vi "Calib_General_Setup.vi"(0 "Ref Instrument type":T1=enum."Generic Polynomial", 1 "Requested No of samples":i32=128 min=0 step=1, 2 "Sampling rate (Hz)":sgl=1000.0 format="%.2f", 5 "2nd ref instrument":T2={"2nd Ref type"=enum."LDA", "2nd inst present"=TRUE}, 9 "Temp":dbl=20.0 format="%.1f", 12 "Abs Press (mbar)":dbl=1005.0 format="%.2f") -> (8 "Output string":string, 10 "LDA Data":bool)   [LabVIEW 2022 SP3]
uses:
  Controls/Ref_Inst_type.ctl
  Controls/Analysis_info_cluster.ctl
  Controls/Inst_type.ctl
  Controls/Instrument_Array.ctl
  Controls/channelState.ctl
  Controls/Graph_Type.ctl
  Globals/Meas_global.vi
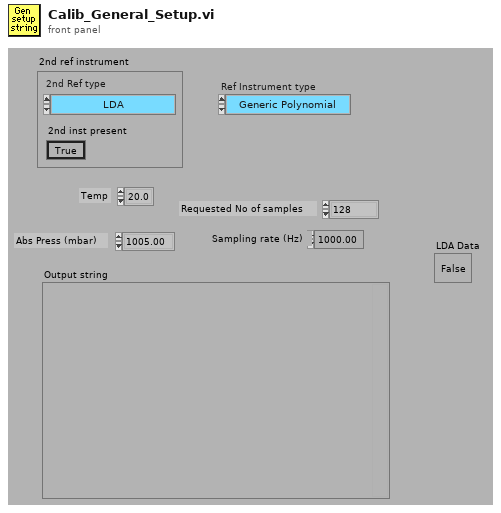
[diagram p1: front panel]
types:
  T1 = typedef "Ref_Inst_type.ctl" = enum16{"Propellor anemometer", "Pressure Transducer", "Raw voltage", "Pitot-static tube", "Generic Linear", "Generic Polynomial", "Thermocouple", "LDA", "Enter Value", "ADAM Channel"}
  T2 = cluster{"2nd Ref type":T1, "2nd inst present":bool}
  T3 = typedef "Analysis_info_cluster.ctl" = cluster{"Colour":u32, "Inst type":T4, "Inst name":string, "Symbol":string, "Code name":string, "Extra Info":string, "Inst Array":T5, "U":dbl, "u^2":dbl, "u^3":dbl, "u^4":dbl, "Skew_u":dbl, "Kurt_u":dbl, "Sd Error in Mean":dbl, "% u'/U":dbl, "X":dbl, "Y":dbl, "Z":dbl, "Timescale integral Estimate":dbl, "Sd Error in Variance":dbl, "Calib File":path, "Calib Constants":dbl[], "Output Position":bool, "Stats":enum16{"None", "Basic", "Full"}, "Av Sampling Rate":dbl, "Av No of Samples":dbl, "Total Meas Time (s)":dbl, "OrigChName":string, "Max value":dbl, "Min value":dbl, "Req Sample Rate Hz":dbl, "Sync Delay Time (s)":dbl, "Ch No":i16, "Device":string, "Use Latest Calib":bool, "Port":string, "Metadata Ch Names":string[], "Metadata Ch Values":string[], "Label":string, "chState":T6, "Point Drift":dbl, "inputConfig":string}
  T4 = typedef "Inst_type.ctl" = enum16{"Raw voltage", "Raw with zero offsetting", "Propeller anemometer", "Pressure Transducer", "Pitot-static tube", "Hot wire", "Cross wire 1", "Cross wire 2", "Generic Linear", "Generic Polynomial", "Generic BackPoly", "Fast FID", "Thermocouple", "Cold wire", "Pulsed Wire", "LDA Vel", "LDA Tran time", "LDA Arr time", "Microphone"}
  T5 = typedef "Instrument_Array.ctl" = enum16{"PWA", "LDA", "Analogue"}
  T6 = typedef "channelState.ctl" = enum32{"No Selection", "Solo", "Mute"}
  T7 = typedef "Graph_Type.ctl" = enum16{"Show no graph", "Voltage trace", "Velocity trace", "Vel histogram", "Spectrum", "f.E(f) v Log f", "Auto-Corr"}
  T8 = cluster{"Plot 1":u16, "Plot 2":u16, "Save graph":u16, "Plot Type":T7}
  T9 = enum16{"From String to Cluster", "From Cluster to String"}
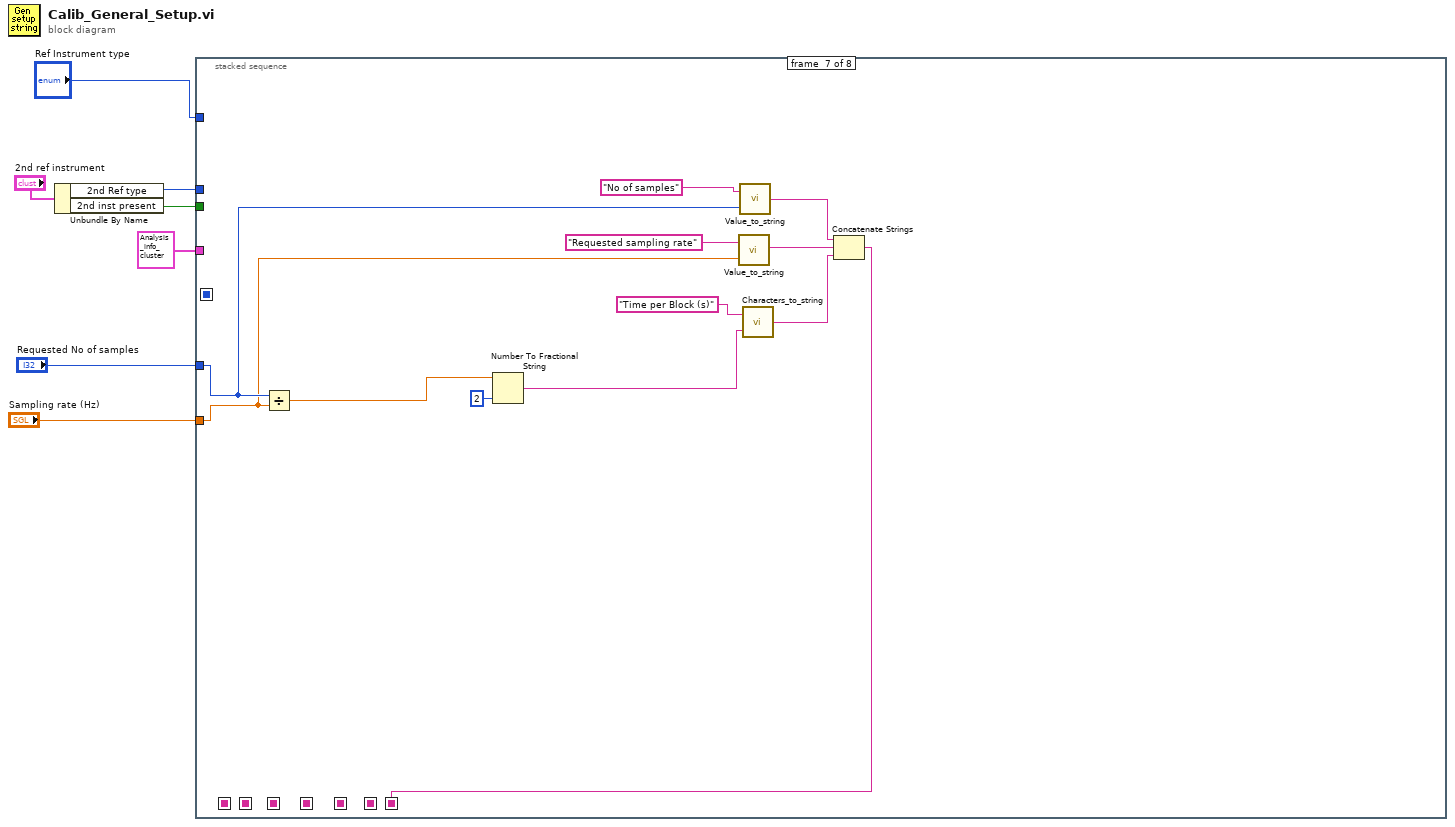
[diagram p0: block diagram]
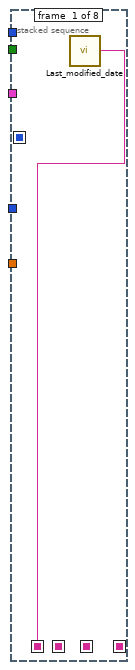
[diagram p2: hidden frame]
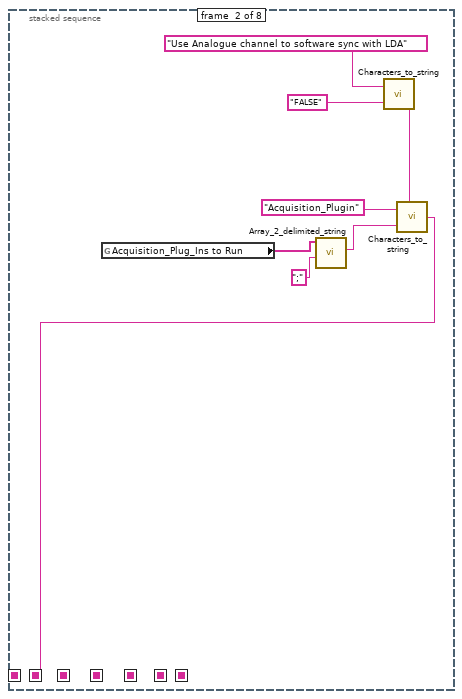
[diagram p3: hidden frame]
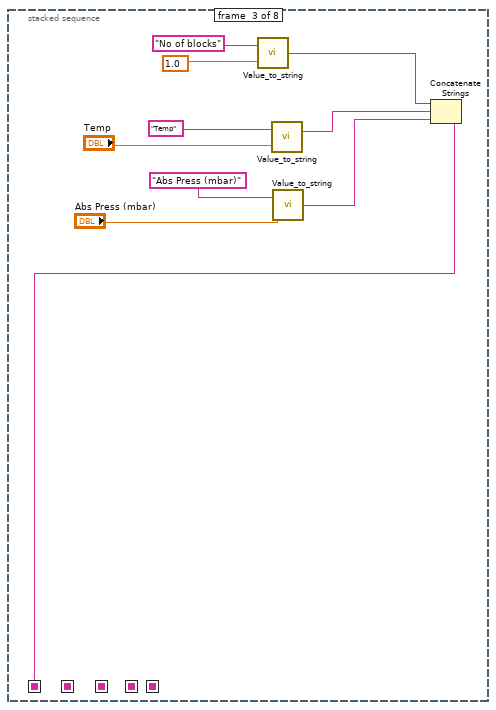
[diagram p4: hidden frame]
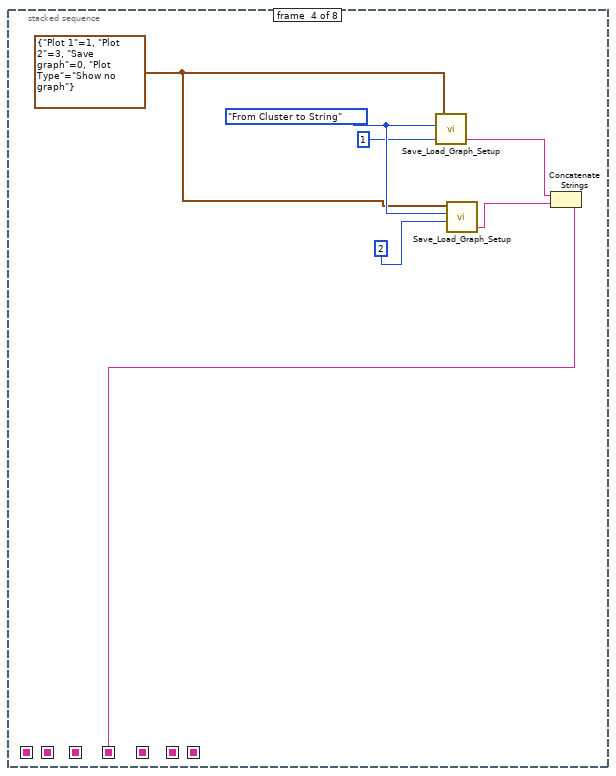
[diagram p5: hidden frame]
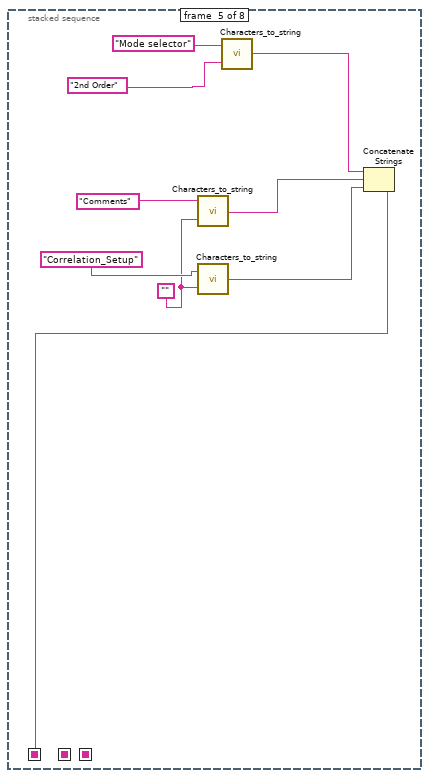
[diagram p6: hidden frame]
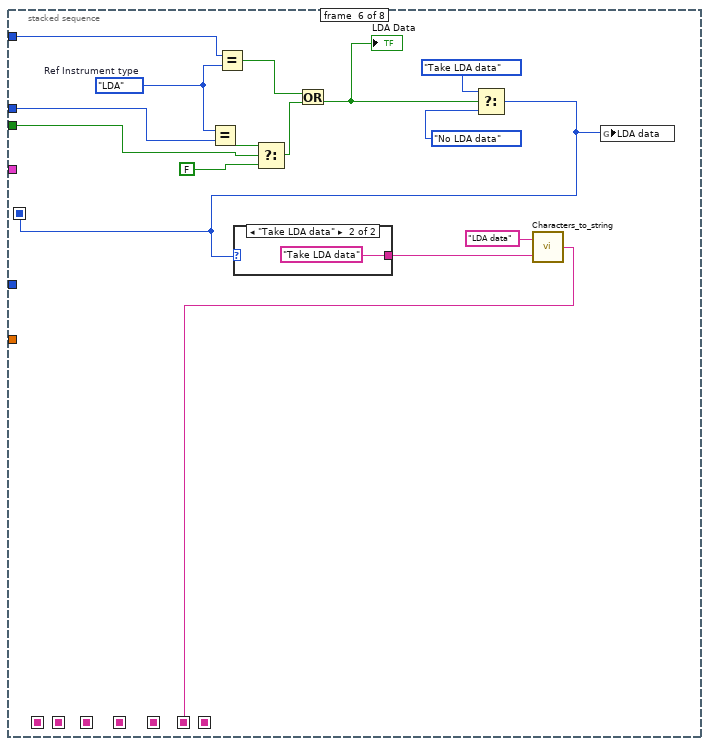
[diagram p7: hidden frame]
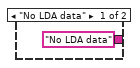
[diagram p8: hidden frame]
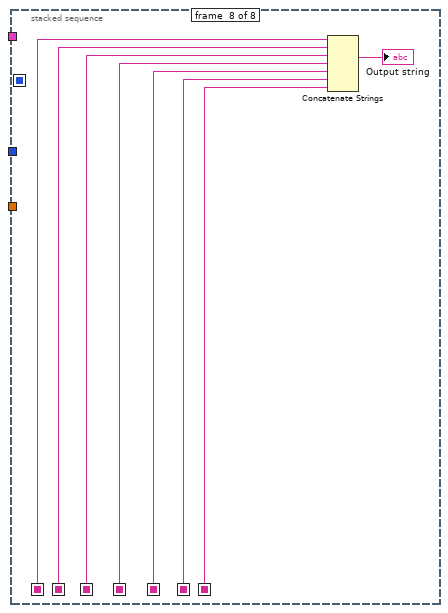
[diagram p9: hidden frame]
diagram:
  n1 = Unbundle By Name("2nd ref instrument") -> ("2nd Ref type"=w5:T1, "2nd inst present"=w4:bool)
  n2 = stacked-sequence {
    seq-local: [_ _ w25 _ _ _ _ _] -> [_ _ _ _ _ _ _ w79]
    seq-local: [_ w9 _ _ _ _ _ _] -> [_ _ _ _ _ _ _ w78]
    seq-local: [_ _ _ _ _ w55 _ _] -> [_ _ _ _ _ _ _ w74]
    seq-local: [_ _ _ _ _ _ w60 _] -> [_ _ _ _ _ _ _ w73]
    seq-local: [_ _ _ w28 _ _ _ _] -> [_ _ _ _ _ _ _ w76]
    seq-local: [_ _ _ _ w37 _ _ _] -> [_ _ _ _ _ _ _ w75]
    seq-local: [w8 _ _ _ _ _ _ _] -> [_ _ _ _ _ _ _ w72]
    seq-local: [_ _ _ _ _ w48 _ _] -> [_ _ _ _ _ _ _ _]
    tunnel: T3 {"Colour"=0, "Inst type"=enum."Pitot-static tube", "Inst name"="Manometer voltage", "Symbol"="U", "Code name"="", "Extra Info"="U", "Inst Array"=enum."PWA", "U"=0.0, "u^2"=0.0, "u^3"=0.0, "u^4"=0.0, "Skew_u"=0.0, "Kurt_u"=0.0, "Sd Error in Mean"=0.0, "% u'/U"=0.0, "X"=0.0, "Y"=0.0, "Z"=0.0, "Timescale integral Estimate"=0.0, "Sd Error in Variance"=0.0, "Calib File"=path "", "Calib Constants"=[], "Output Position"=FALSE, "Stats"=enum."None", "Av Sampling Rate"=0.0, "Av No of Samples"=0.0, "Total Meas Time (s)"=0.0, "OrigChName"="", "Max value"=0.0, "Min value"=0.0, "Req Sample Rate Hz"=0.0, "Sync Delay Time (s)"=0.0, "Ch No"=0, "Device"="", "Use Latest Calib"=FALSE, "Port"="", "Metadata Ch Names"=[], "Metadata Ch Values"=[], "Label"="", "chState"=enum."Solo", "Point Drift"=0.0, "inputConfig"=""} -> [_ _ _ _ _ _ _ _]
    tunnel: "Ref Instrument type" -> [_ _ _ _ _ w45 _ _]
    tunnel: w5 -> [_ _ _ _ _ w44 _ _]
    tunnel: w4 -> [_ _ _ _ _ w43 _ _]
    tunnel: "Requested No of samples" -> [_ _ _ _ _ _ w65 _]
    tunnel: "Sampling rate (Hz)" -> [_ _ _ _ _ _ w64 _]
    frame #0 {
      n3 = call "Last_modified_date.vi"() -> ("concatenatedRevisions"=w8:string)  [unwired: 1 in, 1 out]
    }
    frame #1 {
      n4 = global read "Meas_global.vi" "Acquisition_Plug_Ins to Run"() -> (w12:string[])
      n5 = call "Array_2_delimited_string.vi"("delimiter (Tab)"=";", "Array of Strings"=w12) -> ("delimited string"=w13:string)  [unwired: 9 in]
      n6 = call "Characters_to_string.vi"("Characters to write"="FALSE", "Label for characters"="Use Analogue channel to software sync with LDA") -> ("Output string"=w10:string)  [unwired: 1 in]
      n7 = call "Characters_to_string.vi"("stringIn"=w10, "Characters to write"=w13, "Label for characters"="Acquisition_Plugin") -> ("Output string"=w9:string)
    }
    frame #2 {
      n8 = call "Value_to_string.vi"("Value"=1.0, "Label for value"="No of blocks") -> ("Output string"=w19:string)  [unwired: 1 in]
      n9 = call "Value_to_string.vi"("Value"="Temp", "Label for value"="Temp") -> ("Output string"=w22:string)  [unwired: 1 in]
      n10 = call "Value_to_string.vi"("Value"="Abs Press (mbar)", "Label for value"="Abs Press (mbar)") -> ("Output string"=w21:string)  [unwired: 1 in]
      n11 = Concatenate Strings(w19, w22, w21) -> (w25:string)
    }
    frame #3 {
      w27 = T8 {"Plot 1"=1, "Plot 2"=3, "Save graph"=0, "Plot Type"=enum."Show no graph"} ("Graph in")
      w31 = T9."From Cluster to String" ("Mode")
      n12 = call "Save_Load_Graph_Setup.vi"("Graph Number"=1, "Mode"=w31, "Graph in"=w27) -> ("Setup String Out"=w33:string)  [unwired: 1 in, 2 out]
      n13 = call "Save_Load_Graph_Setup.vi"("Graph Number"=2, "Mode"=w31, "Graph in"=w27) -> ("Setup String Out"=w32:string)  [unwired: 1 in, 2 out]
      n14 = Concatenate Strings(w33, w32) -> (w28:string)
    }
    frame #4 {
      w34 = ""
      n15 = call "Characters_to_string.vi"("Characters to write"=w34, "Label for characters"="Comments") -> ("Output string"=w38:string)  [unwired: 1 in]
      n16 = call "Characters_to_string.vi"("Characters to write"=w34, "Label for characters"="Correlation_Setup") -> ("Output string"=w35:string)  [unwired: 1 in]
      n17 = call "Characters_to_string.vi"("Characters to write"="2nd Order", "Label for characters"="Mode selector") -> ("Output string"=w40:string)  [unwired: 1 in]
      n18 = Concatenate Strings(w40, w38, w35) -> (w37:string)
    }
    frame #5 {
      w47 = Ref_Inst_type."LDA"  # Ref Instrument type
      n19 = Equal?(x=w47, y=w44) -> (x = y?=w54:bool)
      n20 = Equal?(x=w45, y=w47) -> (x = y?=w51:bool)
      n21 = Select(t=w54, s=w43, f=FALSE) -> (s? t:f=w52:bool)
      n22 = Or(x=w51, y=w52) -> (x .or. y?=w46:bool)
      "LDA Data" <- w46
      n23 = Select(t=enum16{"No LDA data", "Take LDA data"}."Take LDA data" ("LDA data"), s=w46, f=enum16{"No LDA data", "Take LDA data"}."No LDA data" ("LDA data")) -> (s? t:f=w48:enum16{"No LDA data", "Take LDA data"})
      n24 = case shown="\"Take LDA data\"" w48 {
        tunnel: ["No LDA data" "Take LDA data"] -> w56
        frame "No LDA data" {
        }
        frame "Take LDA data" {
        }
      }
      n25 = call "Characters_to_string.vi"("Characters to write"=w56, "Label for characters"="LDA data") -> ("Output string"=w55:string)  [unwired: 1 in]
      n26 = global write "Meas_global.vi" "LDA data"(w48) -> ()
    }
    frame #6 {
      n27 = Divide(x=w65, y=w64) -> (x/y=w70:sgl)
      n28 = Number To Fractional String(number=w70, precision (6)=i16 2) -> (F-format string=w68:string)  [unwired: 2 in]
      n29 = call "Value_to_string.vi"("Value"=w64, "Label for value"="Requested sampling rate") -> ("Output string"=w62:string)  [unwired: 1 in]
      n30 = call "Value_to_string.vi"("Value"=w65, "Label for value"="No of samples") -> ("Output string"=w63:string)  [unwired: 1 in]
      n31 = call "Characters_to_string.vi"("Characters to write"=w68, "Label for characters"="Time per Block (s)") -> ("Output string"=w61:string)  [unwired: 1 in]
      n32 = Concatenate Strings(w63, w62, w61) -> (w60:string)
    }
    frame #7 {
      n33 = Concatenate Strings(w72, w78, w79, w76, w75, w74, w73) -> (→"Output string":string)
    }
  }
